vi "Handle Mouse Leave.vi"(8 "error in (no error)":errorcluster, 11 "Toolbar Control in":refnum<class "Toolbar Control.lvclass">) -> (0 "error out":errorcluster, 2 "Toolbar Image":picture, 3 "Toolbar Control out":refnum<class "Toolbar Control.lvclass">)   [LabVIEW 2011, in "Toolbar Control.lvclass"]
doc: "This VI handles the Mouse Leave event on the toolbar. When the Mouse Leave event is detected run this VI.\n\n-------------\nDeveloped by Brian Hoover (hooovahh)"
uses:
  Toolbar Control.lvclass
  Toolbar Control.lvclass/Toolbar Control.ctl
  Controls/Mouse State.ctl
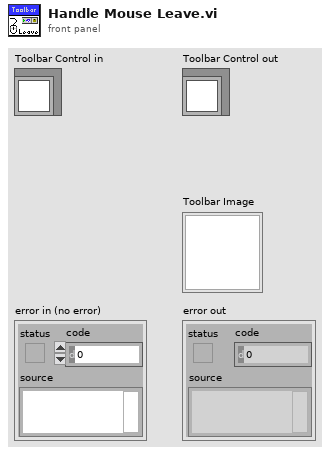
[diagram p1: front panel]
types:
  T1 = typedef "Mouse State.ctl" = enum8{"Normal", "Mouse Over", "Mouse Down"}
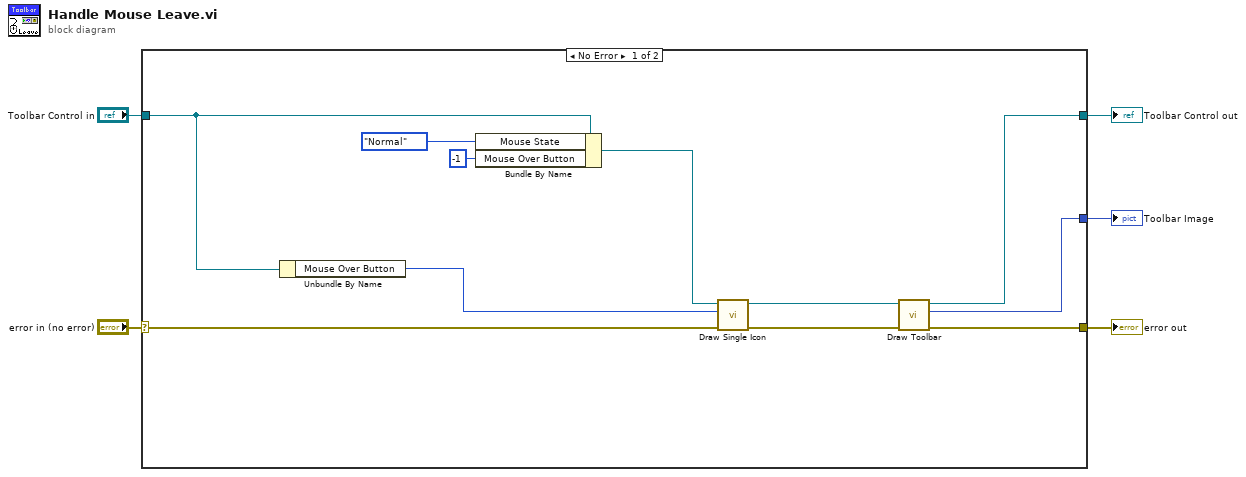
[diagram p0: block diagram]
diagram:
  n1 = case shown="No Error" "error in (no error)" {
    selector: "error in (no error)" -> [w7 w17]
    tunnel: [w14 w18] -> w3
    tunnel: "Toolbar Control in" -> [w16 w18]
    tunnel: [w13 _] -> w2
    tunnel: [w12 w17] -> w1
    frame No Error {
      n2 = Unbundle By Name(w16) -> ("Mouse Over Button"=w6:i32)
      n3 = Bundle By Name(cluster=w16, "Mouse State"=Mouse_State."Normal", "Mouse Over Button"=-1) -> (w15:refnum<class "Toolbar Control.lvclass">)
      n4 = call "Draw Single Icon.vi"("error in (no error)"=w7, "Icon Index"=w6, "Toolbar Control in"=w15) -> ("error out"=w8:errorcluster, "Toolbar Control out"=w9:refnum<class "Toolbar Control.lvclass">)  [unwired: 7 in]
      n5 = call "Draw Toolbar.vi"("error in (no error)"=w8, "Toolbar Control in"=w9) -> ("error out"=w12:errorcluster, "Toolbar Image"=w13:picture, "Toolbar Control out"=w14:refnum<class "Toolbar Control.lvclass">)  [unwired: 7 in]
    }
    frame Error {
    }
  }
  "error out" <- w1
  "Toolbar Control out" <- w3
  "Toolbar Image" <- w2
